vi "KE622x -- 2182 -A Set Range.vi"(0 "622x Resource In":refnum<visa-resource-name>, 1 "Check For SCPI Errors? (T)":bool=TRUE, 7 "2182/2182A Range":enum16{"10mV", "100mV", "1V", "10V", "100V"}(ring), 11 "error in (no error)":errorcluster) -> (4 "622x Resource Out (dupl)":refnum<visa-resource-name>, 15 "error out":errorcluster)   [LabVIEW 2013, in "Keithly user program.lvlib"]
uses:
  Keithly user program.lvlib
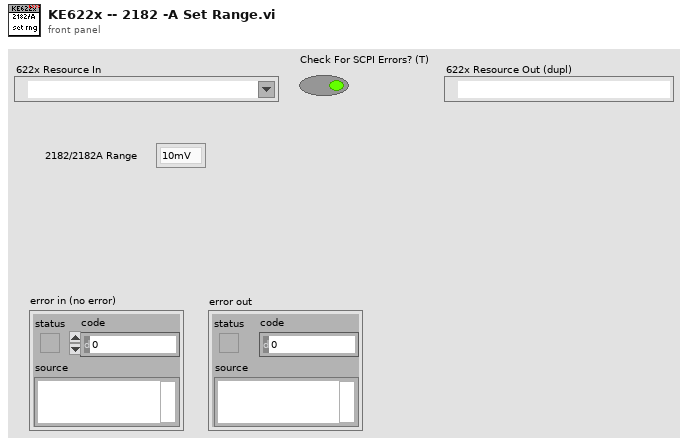
[diagram p1: front panel]
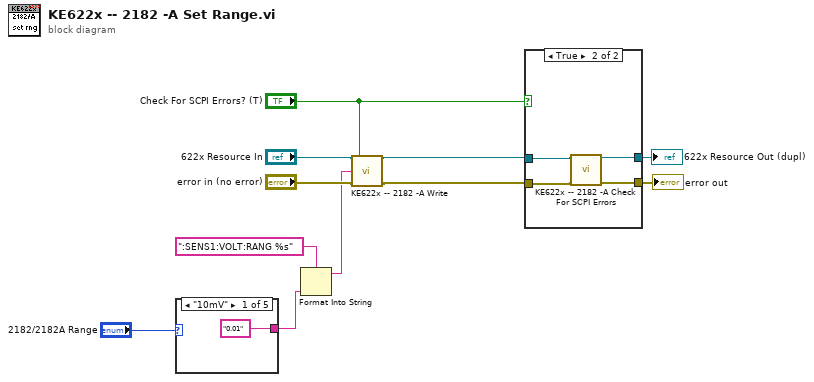
[diagram p0: block diagram]
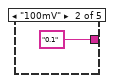
[diagram p2: hidden frame]
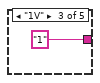
[diagram p3: hidden frame]
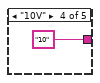
[diagram p4: hidden frame]
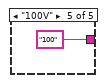
[diagram p5: hidden frame]
diagram:
  n1 = case shown="\"10mV\"" "2182/2182A Range" {
    tunnel: ["0.01" "0.1" "1" "10" "100"] -> w8
    frame "10mV" {
    }
    frame "100mV" {
    }
    frame "1V" {
    }
    frame "10V" {
    }
    frame "100V" {
    }
  }
  n2 = Format Into String(format string=":SENS1:VOLT:RANG %s", w8) -> (resulting string=w2:string)  [unwired: 2 in, 1 out]
  n3 = call "KE622x -- 2182 -A Write.vi"("Resource In"="622x Resource In", "Check For SCPI Errors? (T)"="Check For SCPI Errors? (T)", "2182-A Write String"=w2, "error in (no error)"="error in (no error)") -> ("Resource Out (dupl)"=w5:refnum<visa-resource-name>, "error out"=w1:errorcluster)  [unwired: 10 in]
  n4 = case shown="True" "Check For SCPI Errors? (T)" {
    tunnel: w5 -> [w18 w22]
    tunnel: w1 -> [w17 w20]
    tunnel: [w18 w21] -> w11
    tunnel: [w17 w19] -> w10
    frame False {
    }
    frame True {
      n5 = call "KE622x -- 2182 -A Check For SCPI Errors.vi"("VISA Resource In"=w22, "error in (no error)"=w20) -> ("VISA Resource Out (dupl)"=w21:refnum<visa-resource-name>, "error out"=w19:errorcluster)  [unwired: 10 in, 2 out]
    }
  }
  "622x Resource Out (dupl)" <- w11
  "error out" <- w10
